vi "Pharse_Return (SubVI).vi"(4 "buffer in":string) -> (0 "byte array":u8[](array[numeric]) format="%.0x", 1 "result_content":string, 2 "Err?":bool)   [LabVIEW 8.6]
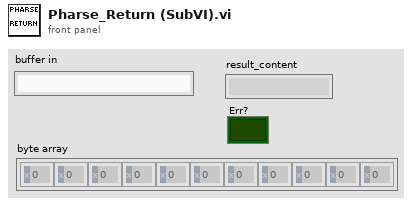
[diagram p1: front panel]
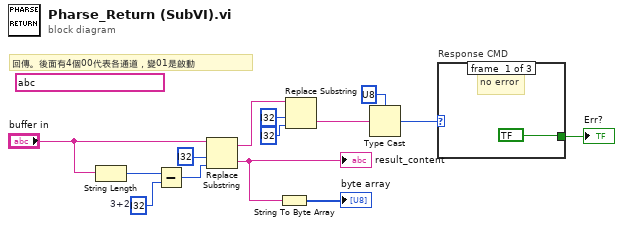
[diagram p0: block diagram]
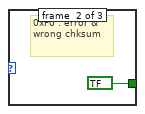
[diagram p2: hidden frame]
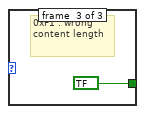
[diagram p3: hidden frame]
diagram:
  (unwired) string ?
  w14 = i32 ?  # 3+2
  # "回傳。後面有4個00代表各通道，變01是啟動"
  n1 = String Length(string="buffer in") -> (length=w13:i32)
  n2 = Subtract(x=w13, y=w14) -> (x-y=w9:i32)
  n3 = Replace Substring(2:w9, 3:i32 ? ("offset (0)"), 5:"buffer in") -> (0:w5:string, 1:w8:string)  [unwired: 1 in]
  "result_content" <- w5
  n4 = String To Byte Array(string=w5) -> (unsigned byte array=→"byte array":u8[])
  n5 = Replace Substring(2:i32 ? ("length (len. of substring)"), 3:i32 ? ("offset (0)"), 5:w8) -> (0:w3:string)  [unwired: 1 in, 1 out]
  n6 = Type Cast(type=u8 ?, x=w3) -> (*(type *) &x=w2:u8)
  n7 = case "Response CMD" shown="241" w2 {
    tunnel: [bool ? bool ? bool ?] -> w1
    frame #0 {
      # "no error"
    }
    frame #1 {
      # "0xF0 : error & \nwrong chksum"
    }
    frame #2 {
      # "0xF1 : wrong \ncontent length"
    }
  }
  "Err?" <- w1
